vi "check_folder_no_prompt (SubVI).vi"(11 "path in":path) -> (3 "path out":path)   [LabVIEW 2018]
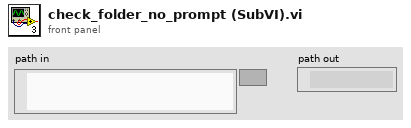
[diagram p1: front panel]
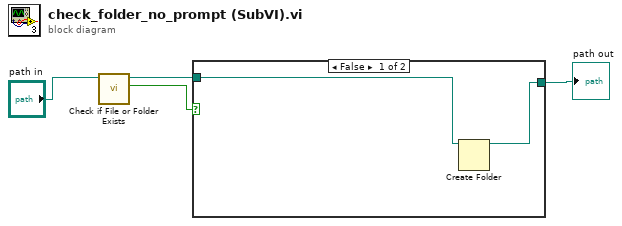
[diagram p0: block diagram]
diagram:
  n1 = call <vilib>:"Check if File or Folder Exists.vi"("path"="path in") -> ("file or folder exists?"=w2:bool, "dup path"=w1:path)  [unwired: 8 in, 1 out]
  n2 = case shown="False" w2 {
    tunnel: w1 -> [w6 w7]
    tunnel: [w5 w7] -> w4
    frame False {
      n3 = Create Folder(path (use dialog)=w6) -> (created path=w5:path)  [unwired: 2 in, 2 out]
    }
    frame True {
    }
  }
  "path out" <- w4
